vi "neuron.vi"(8 "opinons":dbl[](array[numeric]), 11 "inputs":dbl[][](array[numeric])) -> (2 "output":dbl[](array[numeric]))   [LabVIEW 2014]
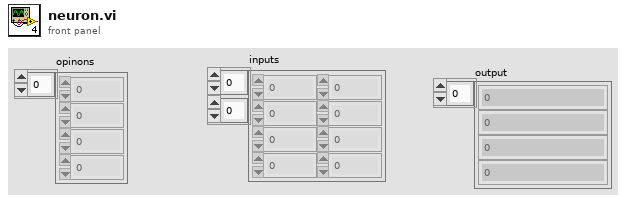
[diagram p1: front panel]
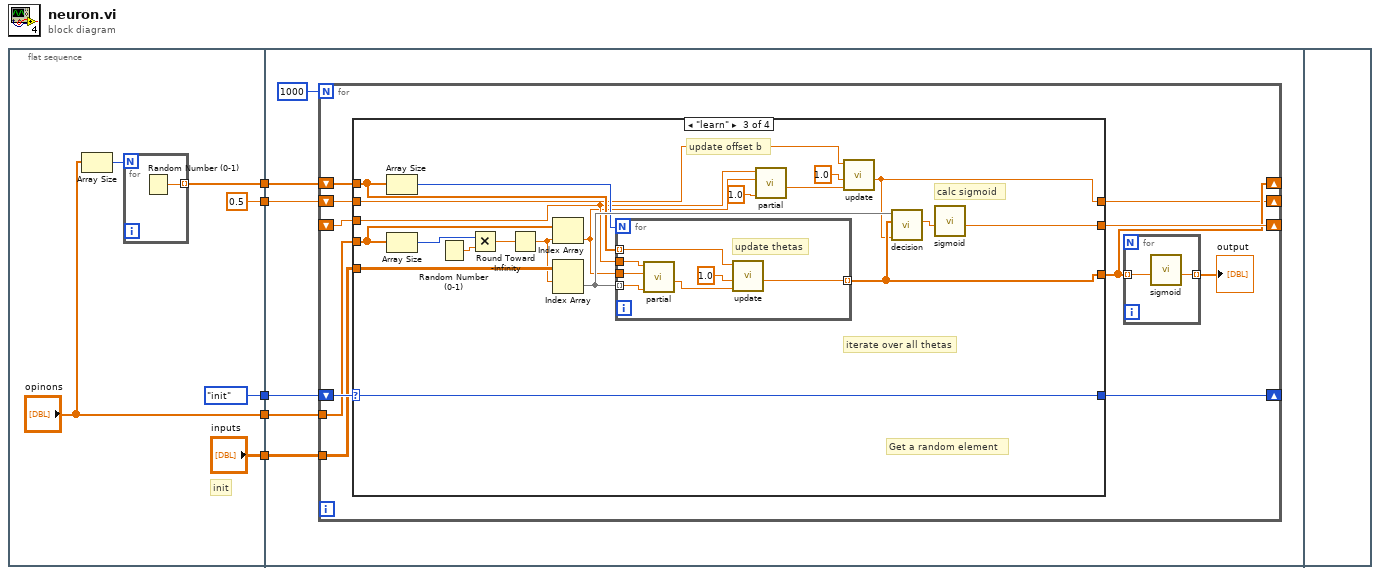
[diagram p0: block diagram]
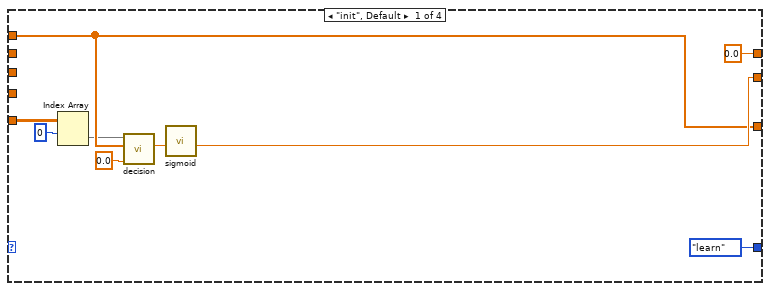
[diagram p2: hidden frame]
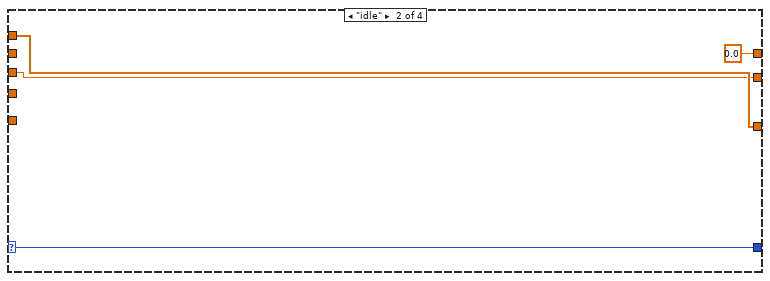
[diagram p3: hidden frame]
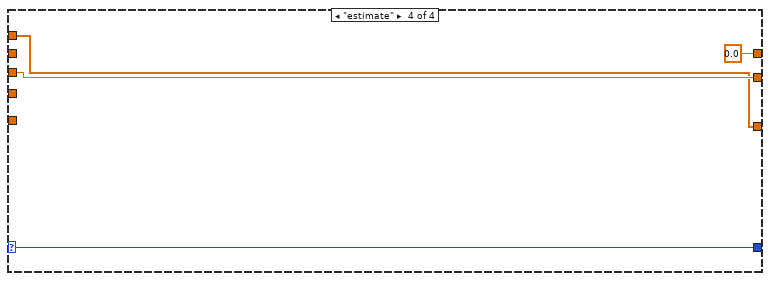
[diagram p4: hidden frame]
diagram:
  n1 = flat-sequence {
    tunnel: [enum16{"init", "idle", "learn", "estimate"}."init"] -> w5
    tunnel: ["inputs"] -> w4
    tunnel: ["opinons"] -> w3
    tunnel: [0.5] -> w2
    tunnel: [w6] -> w1
    tunnel: w5 -> [w18]
    tunnel: w4 -> [w14]
    tunnel: w3 -> [w16]
    tunnel: w2 -> [w13]
    tunnel: w1 -> [w15]
    frame #0 {
      # "init"
      n2 = Array Size(array="opinons") -> (size(s)=w7:i32)
      n3 = for {
        N: w7 -> [_]
        tunnel: [w12] -> w6 mode=indexing
        n4 = Random Number (0-1)() -> (number: 0 to 1=w12:dbl)
      }
    }
    frame #1 {
      n5 = for {
        N: 1000 -> [_]
        shift-right: [w29] -> _
        shift-left: _ -> [w28]
        shift-right: [w27] -> _
        shift-left: w18 -> [w26]
        tunnel: w16 -> [w25]
        shift-right: [w21] -> _
        shift-left: w15 -> [w24]
        tunnel: w14 -> [w23]
        shift-right: [w19] -> _
        shift-left: w13 -> [w20]
        n6 = case shown="\"learn\"" w26 {
          selector: w26 -> [_ w42 w45 w73]
          tunnel: [w39 w43 w57 w75] -> w29
          tunnel: w28 -> [_ w43 w51 w75]
          tunnel: [enum16{"init", "idle", "learn", "estimate"}."learn" w42 w45 w73] -> w27
          tunnel: w24 -> [w35 w44 w55 w74]
          tunnel: w23 -> [w36 _ w61 _]
          tunnel: w25 -> [_ _ w62 _]
          tunnel: [w35 w44 w58 w74] -> w21
          tunnel: w20 -> [_ _ w48 _]
          tunnel: [0.0 ("X'") 0.0 ("X'") w46 0.0 ("X'")] -> w19
          frame "init", Default {
            n7 = Index Array(array=w36, index (row)=0) -> (element=w33:dbl[])  [unwired: 1 in]
            n8 = call "decision.vi"("offset"=0.0, "weights"=w35, "inputs"=w33) -> ("decision"=w40:dbl)  [unwired: 8 in]
            n9 = call "sigmoid.vi"("t"=w40) -> ("S(t)"=w39:dbl)  [unwired: 10 in]
          }
          frame "idle" {
          }
          frame "learn" {
            # "iterate over all thetas"
            # "Get a random element"
            # "calc sigmoid"
            # "update offset b"
            n10 = Array Size(array=w55) -> (size(s)=w56:i32)
            n11 = Array Size(array=w62) -> (size(s)=w64:i32)
            n12 = Random Number (0-1)() -> (number: 0 to 1=w63:dbl)
            n13 = Multiply(x=w64, y=w63) -> (x*y=w54:dbl)
            n14 = Round Toward -Infinity(1:w54) -> (0:w53:dbl)
            n15 = Index Array(array=w62, index=w53) -> (element=w50:dbl)
            n16 = Index Array(array=w61, index (row)=w53) -> (element=w59:dbl[])  [unwired: 1 in]
            n17 = for {
              N: w56 -> [_]
              tunnel: w51 -> [w69]
              tunnel: w55 -> [w68] mode=indexing
              tunnel: [w67] -> w58 mode=indexing
              tunnel: w59 -> [w66] mode=indexing
              tunnel: w50 -> [w65]
              # "update thetas"
              n18 = call "partial.vi"("input"=w66, "opinon"=w65, "sigmoid g(~)"=w69) -> ("deltaX"=w70:dbl)  [unwired: 8 in]
              n19 = call "update.vi"("deltaX"=w70, "Alpha"=1.0, "X"=w68) -> ("X'"=w67:dbl)  [unwired: 8 in]
            }
            n20 = call "partial.vi"("input"=1.0, "opinon"=w50, "sigmoid g(~)"=w51) -> ("deltaX"=w49:dbl)  [unwired: 8 in]
            n21 = call "update.vi"("deltaX"=w49, "Alpha"=1.0, "X"=w48) -> ("X'"=w46:dbl)  [unwired: 8 in]
            n22 = call "decision.vi"("offset"=w46, "weights"=w58, "inputs"=w59) -> ("decision"=w60:dbl)  [unwired: 8 in]
            n23 = call "sigmoid.vi"("t"=w60) -> ("S(t)"=w57:dbl)  [unwired: 10 in]
          }
          frame "estimate" {
          }
        }
        n24 = for {
          tunnel: [w31] -> w22 mode=indexing
          tunnel: w21 -> [w30] mode=indexing
          n25 = call "sigmoid.vi"("t"=w30) -> ("S(t)"=w31:dbl)  [unwired: 10 in]
        }
        "output" <- w22
      }
    }
    frame #2 {
    }
  }
